vi "1.vi"() -> ()   [LabVIEW 2017]
panel:
  out "最大心率":dbl
  in  "年龄":dbl
  in  "枚举":enum16{"女", "男"}(ring)
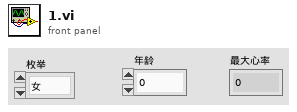
[diagram p1: front panel]
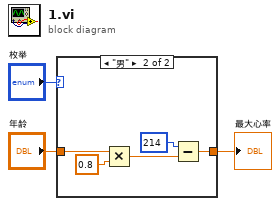
[diagram p0: block diagram]
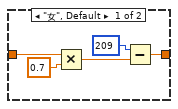
[diagram p2: hidden frame]
diagram:
  n1 = case shown="\"男\"" "枚举" {
    tunnel: "年龄" -> [w7 w10]
    tunnel: [w4 w9] -> w1
    frame "女", Default {
      n2 = Multiply(x=w7, y=0.7) -> (x*y=w5:dbl)
      n3 = Subtract(x=209, y=w5) -> (x-y=w4:dbl)
    }
    frame "男" {
      n4 = Multiply(x=w10, y=0.8) -> (x*y=w11:dbl)
      n5 = Subtract(x=214, y=w11) -> (x-y=w9:dbl)
    }
  }
  "最大心率" <- w1
